vi "queryMeasureName.vi"(8 "error in (no error)":errorcluster caption="错误输入（无错误）", 10 "Channel":string="1", 11 "N5230 输入":refnum<class "N5230.lvclass"> caption="DNL_LabVIEW Object in") -> (0 "error out":errorcluster caption="错误输出", 1 "Parameter item":string[](array[string]), 2 "Name list":string[](array[string]), 3 "N5230 输出":refnum<class "N5230.lvclass"> caption="DNL_LabVIEW Object out")   [LabVIEW 2011, in "N5230.lvclass"]
uses:
  N5230.lvclass
  N5230.lvclass/N5230.ctl
panel:
  out "Read buffer":string
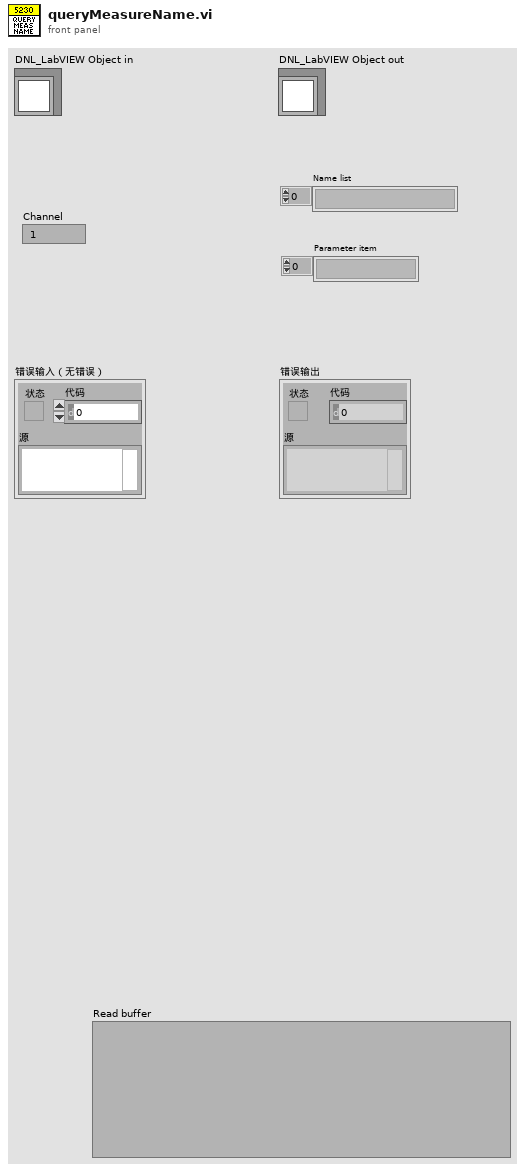
[diagram p1: front panel]
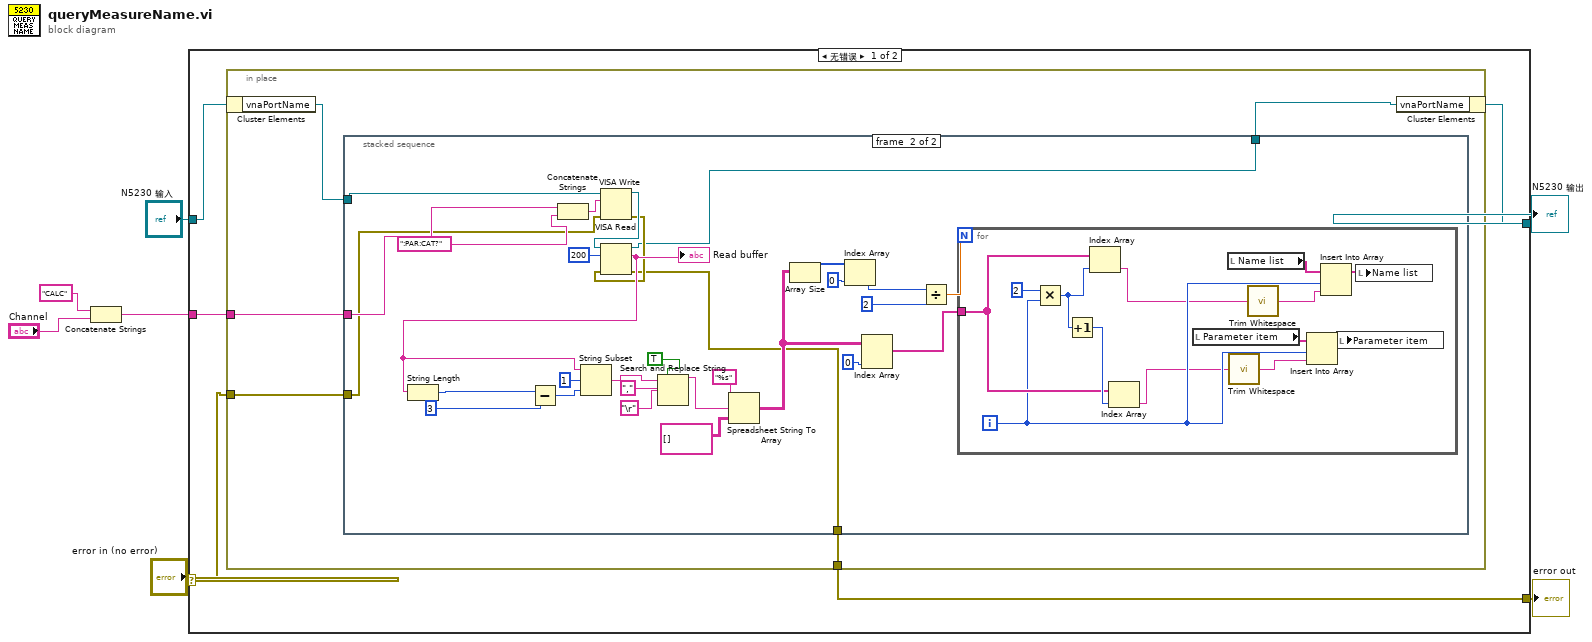
[diagram p0: block diagram]
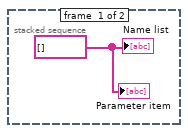
[diagram p2: hidden frame]
diagram:
  n1 = Concatenate Strings("CALC" ("字符串"), "Channel") -> (w1:string)
  n2 = case shown="无错误" "error in (no error)" {
    selector: "error in (no error)" -> [w9 w62]
    tunnel: "N5230 输入" -> [w12 w63]
    tunnel: [w11 w63] -> w5
    tunnel: [w8 w62] -> w4
    tunnel: w1 -> [w10 _]
    frame No Error {
      n3 = in-place {
        in-place-border: w10 -> [w16]
        in-place-border: w9 -> [w15]
        in-place-border: [w14] -> w8
        n4 = in-place-cluster #1(w12) -> ("vnaPortName"=w17:refnum<visa-resource-name>)
        n5 = stacked-sequence {
          tunnel: w17 -> [_ w24]
          tunnel: w16 -> [_ w23]
          tunnel: w15 -> [_ w22]
          tunnel: [_ w20] -> w14
          tunnel: [_ w19] -> w13
          frame #0 {
            w18 = string[] [] ("Name list")
            "Name list" <- w18
            "Parameter item" <- w18
          }
          frame #1 {
            n6 = Concatenate Strings(w23, ":PAR:CAT?") -> (w47:string)
            n7 = VISA Write(VISA resource name=w24, write buffer=w47, error in (no error)=w22) -> (VISA resource name out=w45:refnum<visa-resource-name>, error out=w21:errorcluster)  [unwired: 1 out]
            n8 = VISA Read(VISA resource name=w45, byte count=u32 200, error in (no error)=w21) -> (VISA resource name out=w19:refnum<visa-resource-name>, read buffer=w46:string, error out=w20:errorcluster)  [unwired: 1 out]
            "Read buffer" <- w46
            n9 = String Length(string=w46) -> (length=w32:i32)
            n10 = Subtract(x=w32, y=3) -> (x-y=w34:i32)
            n11 = String Subset(string=w46, offset (0)=1, length (rest)=w34) -> (substring=w35:string)
            n12 = Search and Replace String(replace all?=TRUE ("replace all? (F)"), input string=w35, search string=",", replace string="\r") -> (result string=w27:string)  [unwired: 4 in, 3 out]
            n13 = Spreadsheet String To Array(format string="%s", spreadsheet string=w27, array type (2D Dbl)=string[][] [] ("array 2")) -> (array=w38:string[][])  [unwired: 1 in]
            n14 = Array Size(array=w38) -> (size(s)=w36:i32[])
            n15 = Index Array(array=w36, index=0) -> (element=w41:i32)
            n16 = Index Array(array=w38, index (col)=0 ("disabled index (col)")) -> (element=w40:string[])  [unwired: 1 in]
            n17 = Divide(x=w41, y=2) -> (x/y=w43:dbl)
            n18 = for {
              N: w43 -> [_]
              tunnel: w40 -> [w56]
              i -> [w55]
              n19 = Multiply(x=2, y=w55) -> (x*y=w58:i32)
              n20 = Increment(x=w58) -> (x+1=w57:i32)
              n21 = Index Array(array=w56, index=w58) -> (element=w50:string)
              n22 = Index Array(array=w56, index=w57) -> (element=w52:string)
              n23 = local read "Parameter item"() -> (w54:string[])
              n24 = local read "Name list"() -> (w59:string[])
              n25 = call <vilib>:"Trim Whitespace.vi"("string"=w52) -> ("trimmed string"=w51:string)  [unwired: 1 in]
              n26 = call <vilib>:"Trim Whitespace.vi"("string"=w50) -> ("trimmed string"=w49:string)  [unwired: 1 in]
              n27 = Insert Into Array(array=w54, index=w55, new element=w51) -> (w53:string[])
              n28 = Insert Into Array(array=w59, index=w55, new element=w49) -> (w60:string[])
              n29 = local write "Parameter item"(w53) -> ()
              n30 = local write "Name list"(w60) -> ()
            }
          }
        }
        n31 = in-place-cluster #1("vnaPortName"=w13) -> (w11:refnum<class "N5230.lvclass">)
      }
    }
    frame Error {
    }
  }
  "error out" <- w4
  "N5230 输出" <- w5
